vi "ReadDataFromTDMS.vi"(9 "结束时间":timestamp=timestamp(3517116532.858421 s since 1904-01-01) format="%<%H:%M:%S\n%x>T", 10 "起始时间":timestamp=timestamp(3517116513.32069 s since 1904-01-01) format="%<%H:%M:%S\n%x>T", 11 "通道名":string="声发射") -> (3 "波形图":dbl[](graph))   [LabVIEW 2014]
panel:
  out "大小 2":i32
  out "大小":i32[](array[numeric])
  out "输出数组":dbl[](array[numeric])
  out "错误输出":errorcluster
  out "时间":timestamp[](array[timestamp])
  out "数据":dbl[][](array[numeric])
  in  "文件名":string="data"
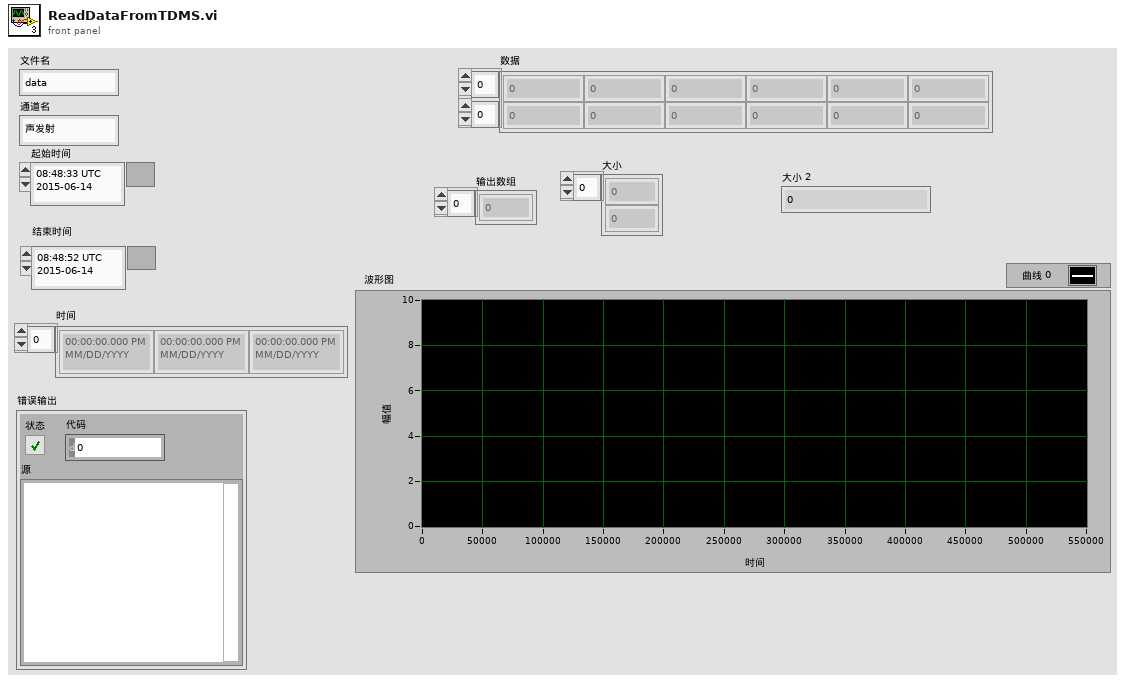
[diagram p1: front panel]
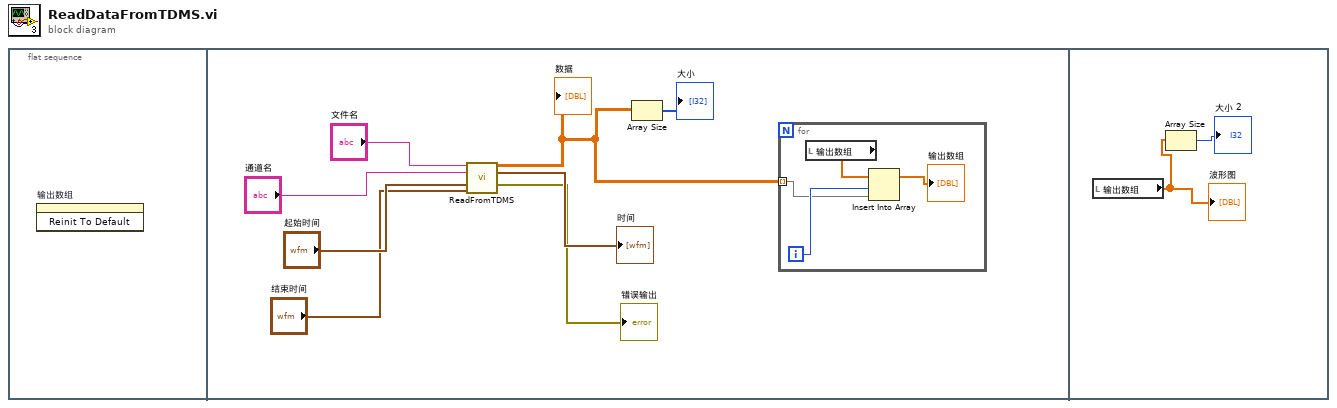
[diagram p0: block diagram]
diagram:
  n1 = flat-sequence {
    frame #0 {
      n2 = invoke on="输出数组" class="Arr (严格)" method="Reinit To Default"() -> ()  [unwired: 3 in, 3 out]
    }
    frame #1 {
      n3 = call "ReadFromTDMS.vi"("文件名"="文件名", "通道名"="通道名", "起始时间"="起始时间", "结束时间"="结束时间") -> ("数据"=w2:dbl[][], "时间"=→"时间":timestamp[], "错误输出"=→"错误输出":errorcluster)  [unwired: 9 in]
      "数据" <- w2
      n4 = Array Size(array=w2) -> (size(s)=→"大小":i32[])
      n5 = for {
        tunnel: w2 -> [w11] mode=indexing
        i -> [w12]
        n6 = local read "输出数组"() -> (w10:dbl[])
        n7 = Insert Into Array(array=w10, index=w12, new element=w11) -> (→"输出数组":dbl[])
      }
    }
    frame #2 {
      n8 = local read "输出数组"() -> (w14:dbl[])
      "波形图" <- w14
      n9 = Array Size(array=w14) -> (size(s)=→"大小 2":i32)
    }
  }
